vi "TDMSLogger_Init.vi"(0 "object in":refnum<class "TDMSLogger.lvclass">, 5 "error in (no error)":errorcluster) -> (14 "object out":refnum<class "TDMSLogger.lvclass">, 16 "cancelled":bool, 19 "error out":errorcluster)   [LabVIEW 2019, in "TDMSLogger.lvclass"]
uses:
  TDMSLogger.lvclass
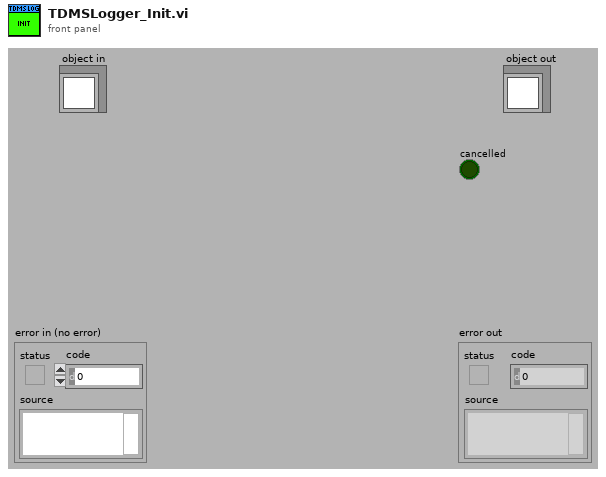
[diagram p1: front panel]
types:
  T1 = enum16{"open", "open or create", "create or replace", "create", "open (read-only)"}
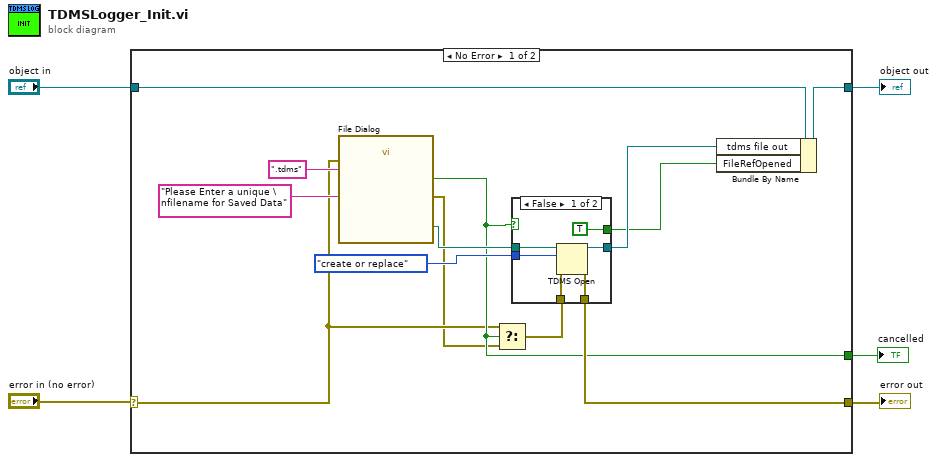
[diagram p0: block diagram]
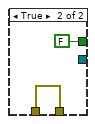
[diagram p2: hidden frame]
diagram:
  n1 = case shown="No Error" "error in (no error)" {
    selector: "error in (no error)" -> [w8 w27]
    tunnel: "object in" -> [w18 w28]
    tunnel: [w17 w28] -> w4
    tunnel: [w16 w27] -> w2
    tunnel: [w9 _] -> w1
    frame No Error {
      n2 = call "File Dialog"("prompt"="Please Enter a unique \nfilename for Saved Data", "error in"=w8, "pattern (all files)"=".tdms") -> ("selected path"=w15:path, "cancelled"=w9:bool, "error out"=w7:errorcluster)  [unwired: 9 in, 1 out]
      n3 = Select(t=w8, s=w9, f=w7) -> (s? t:f=w6:errorcluster)
      n4 = case shown="False" w9 {
        tunnel: [w24 w26] -> w16
        tunnel: w15 -> [w23 _]
        tunnel: [w22 _] -> w14
        tunnel: T1."create or replace" ("operation (0:open)") -> [w21 _]
        tunnel: w6 -> [w20 w26]
        tunnel: [TRUE FALSE] -> w10
        frame False {
          n5 = TDMS Open(8:w20, 10:w21, 11:w23) -> (0:w24:errorcluster, 3:w22:refnum<k34>)  [unwired: 4 in]
        }
        frame True {
        }
      }
      n6 = Bundle By Name(cluster=w18, "tdms file out"=w14, "FileRefOpened"=w10) -> (w17:refnum<class "TDMSLogger.lvclass">)
    }
    frame Error {
    }
  }
  "object out" <- w4
  "error out" <- w2
  "cancelled" <- w1
